vi "Read multiplier.vi"(8 "error in (no error)":errorcluster, 11 "DAQmxTaskAICurrent_General in":refnum<class "DAQmxTaskAICurrent_General.lvclass">) -> (0 "error out":errorcluster, 2 "multiplier":dbl, 3 "DAQmxTaskAICurrent_General out":refnum<class "DAQmxTaskAICurrent_General.lvclass">)   [LabVIEW 2018, in "DAQmxTaskAICurrent_General.lvclass"]
uses:
  DAQmxTaskAICurrent_General.lvclass
  DAQmxTaskAICurrent_General.lvclass/DAQmxTaskAICurrent_General.ctl
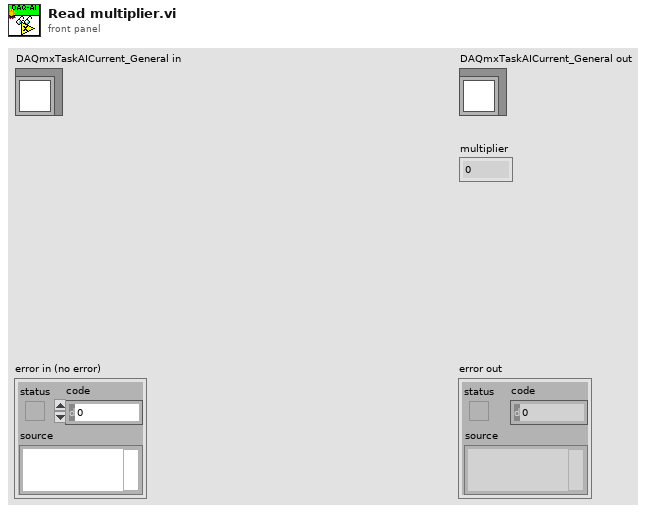
[diagram p1: front panel]
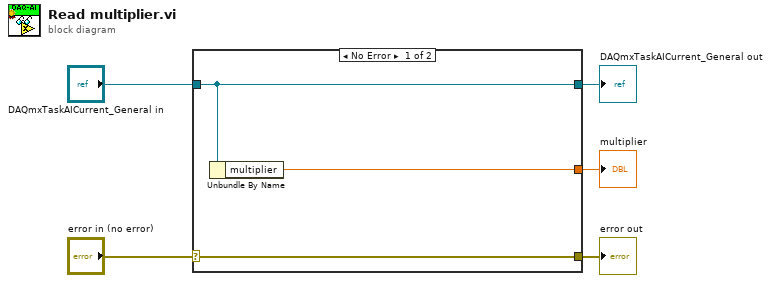
[diagram p0: block diagram]
diagram:
  n1 = case shown="No Error" "error in (no error)" {
    selector: "error in (no error)" -> [w8 w9]
    tunnel: [w8 w9] -> w4
    tunnel: [w7 w10] -> w2
    tunnel: "DAQmxTaskAICurrent_General in" -> [w7 w10]
    tunnel: [w6 _] -> w1
    frame No Error {
      n2 = Unbundle By Name(w7) -> ("multiplier"=w6:dbl)
    }
    frame Error {
    }
  }
  "error out" <- w4
  "DAQmxTaskAICurrent_General out" <- w2
  "multiplier" <- w1
